vi "CCF (SubVI).vi"(1 "Cycling\ntemperature":u16, 2 "N cycles":dbl, 3 "Time cell\nnot used(months)":dbl, 4 "temperature(ªC)":dbl) -> (0 "capacity correction factor":dbl)   [LabVIEW 2017]
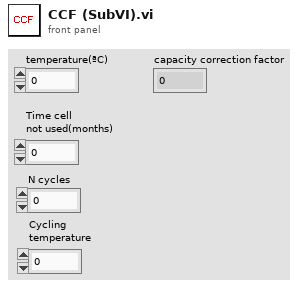
[diagram p1: front panel]
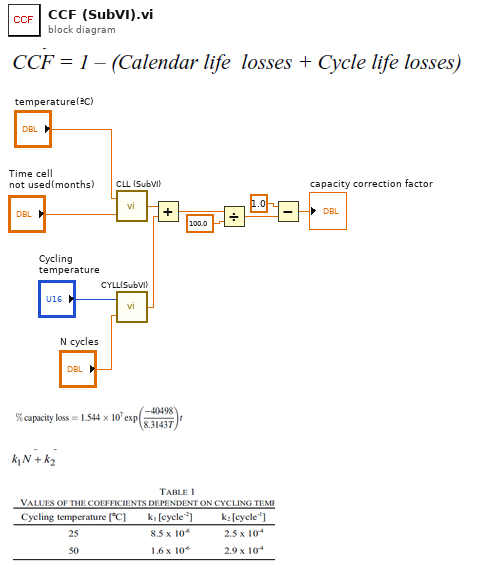
[diagram p0: block diagram]
diagram:
  n1 = call "CLL (SubVI).vi"("Time cell\nnot used(months)"="Time cell\nnot used(months)", "temperature IN"="temperature(ªC)") -> ("calendar life losses(%)"=w6:dbl)
  n2 = call "CYLL(SubVI).vi"("N cycles"="N cycles", "Cycling\ntemperature"="Cycling\ntemperature") -> ("cycle life losses(%)"=w7:dbl)
  n3 = Add(x=w6, y=w7) -> (x+y=w3:dbl)
  n4 = Divide(x=w3, y=100.0) -> (x/y=w1:dbl)
  n5 = Subtract(x=1.0, y=w1) -> (x-y=→"capacity correction factor":dbl)
